vi "nanocal -- nuclear schottky fit V1.vi"() -> ()   [LabVIEW 2020]
uses:
  filename-pattern.ctl
  show-win- control.ctl
  cursor winow.ctl
  cursor window action.ctl
  publisher action.ctl
  3-lorentzian-heat-response action.ctl
  cursor action.ctl
  2Dwindow.ctl
  file -- read-write control.ctl
  array -- freq-voltage transformations action.ctl
  KM_file -- read-write control.ctl
  filename-action.ctl
  9f1323b6-517a-3445-a4b9-7a47222562ae.vi
  3-lorentzian-heat-response.vi/142dd4c5-f9ed-c64b-bc14-a88e3e2c450a.vi
  <vilib>/Analysis/baseanly.llb/A x B.vi
  <vilib>/Analysis/baseanly.llb/Complex A x B.vi
  Q -- check range -- i -- real.vi
  line -- complex.vi
  Q -- check range -- i -- integer.vi
  array -- freq-voltage transformations.vi/05c44075-957c-bc42-b6fa-2799d0bc0485.vi
  Q - not nan -- real.vi
  Q - not nan -- integer.vi
  <vilib>/Array/Sort 2D Array - Pop Stack.vi
  <vilib>/Array/Sort 2D Array - Push Stack.vi
  array -- freq-voltage transformations.vi/05c44075-957c-bc42-b6fa-2799d0bc0485.vi/5dd0d2be-718e-c148-b8fa-e083cdba2843.vi
  array -- freq-voltage transformations.vi/05c44075-957c-bc42-b6fa-2799d0bc0485.vi/095795a0-771d-c341-9fed-d90d2e44c51c.vi
  <vilib>/Analysis/Matrix/Numeric/Conversions/Array To Matrix.vi
  <vilib>/Analysis/Matrix/Numeric/Conversions/Array To Matrix - RA2.vi
  <vilib>/Analysis/baseanly.llb/Inverse Matrix.vi
  <vilib>/Analysis/baseanly.llb/Real Inverse Matrix.vi
  <vilib>/Analysis/polynomials.llb/Multiply Polynomials.vi
  <vilib>/Analysis/polynomials.llb/Multiply Polynomials (DBL).vi
  <vilib>/Analysis/polynomials.llb/Polynomial Roots.vi
  <vilib>/Analysis/polynomials.llb/Polynomial Roots (DBL).vi
  <vilib>/Comparison/Less/Less Functor/Less Functor.lvclass
  server talkto message type.ctl
panel:
  in  "T (K)":dbl=0.001 format="%#_10f"
  out "Plot:  colors":cluster{"Freq out (Hz)":dbl[], dbl[]}[](graph)
  out "String":string
  in  "omega range min (Hz)":dbl=0.001 format="%#_10f"
  in  "omega range max (Hz)":dbl=10000.0 format="%#_10f"
  in  "number of freq points":i32=500
  in  "kappa0":dbl(slide)=5.58e-10 min=0.0 max=0.3 step=1e-12 scale=1e-10..1e-06 scale format="%#_3p"
  in  "tauC":dbl(slide)=0.0059759999999999995 min=0.0 max=0.3 step=1e-06 scale=0.001..10.0 scale format="%#_3p"
  in  "tauN":dbl(slide)=2.349673 min=0.0 max=0.3 step=1e-06 scale=0.001..10.0 scale format="%#_3p"
  in  "tauS":dbl(slide)=0.24445899999999998 min=0.0 max=0.3 step=1e-06 scale=0.001..10.0 scale format="%#_3p"
  in  "T1":dbl(slide)=0.26762 min=0.0 max=0.3 step=1e-06 scale=0.001..10.0 scale format="%#_3p"
  in  "zeta":dbl(slide)=0.23496699999999998 min=0.0 max=0.3 step=1e-06 scale=0.01..10.0 scale format="%#_3p"
  in  "scale gauge: Plot: complex plane":dbl(slide)=625294874.6755459 min=0.0 max=0.3 step=1e-06 scale=1e-05..5000000000.0 scale format="%#_3p"
  in  "Read from file :l":bool
  in  "tr":T1(ring)
  in  "Read from file":path=path "/opt/new/Dropbox/shared_AkashAndreas/paper-CeCoIn5/labviewreadydata/CeCoIn5_2nd_071_12T_0.120K_90deg_fdep_labview_.dat"
  in  "sweeper panel":T2(tab)
  in  ":sweep is ON":bool
  in  "win":T3={"cen (Hz)"=21978.24682616816, "win (Hz)"=4484.832860239923, "left (Hz)"=19735.8303960482, "right (Hz)"=24220.66325628812}
  out "Plot: sweep window":cluster{"Freq out (Hz)":dbl[], dbl[]}[](graph)
  in  "subtract bgnd!":bool
  in  "fit!":bool=TRUE
  in  "cursor window":T4={"left"=19735.8303960482, "right "=24220.66325628812, "center"=21978.24682616816, "window"=4484.832860239923, "cursors"=[0, 1, 2], "relative"=0, "absolute"=0, "fixed vertical offset"=0.0, "vertical offset"=0.0, "skew"=0.0, "default window frac"=0.1, "kind"=enum."symmetric", "skew.left"=0.5, "skew.right"=0.5, "Plot ref"=refnum, "wing order"=enum."forw"}
  in  "save data":enum32{"save/read"}(tab)
  in  "Save to file :s":bool
  in  "Freq sweep name template":T5={"prefix"="RuCl3-rod", "group"="f"}
  in  "Save folder":path=path "/opt/data"
  in  "freq sweep file name":string="f004_RuCl3-rod_060221.dat"
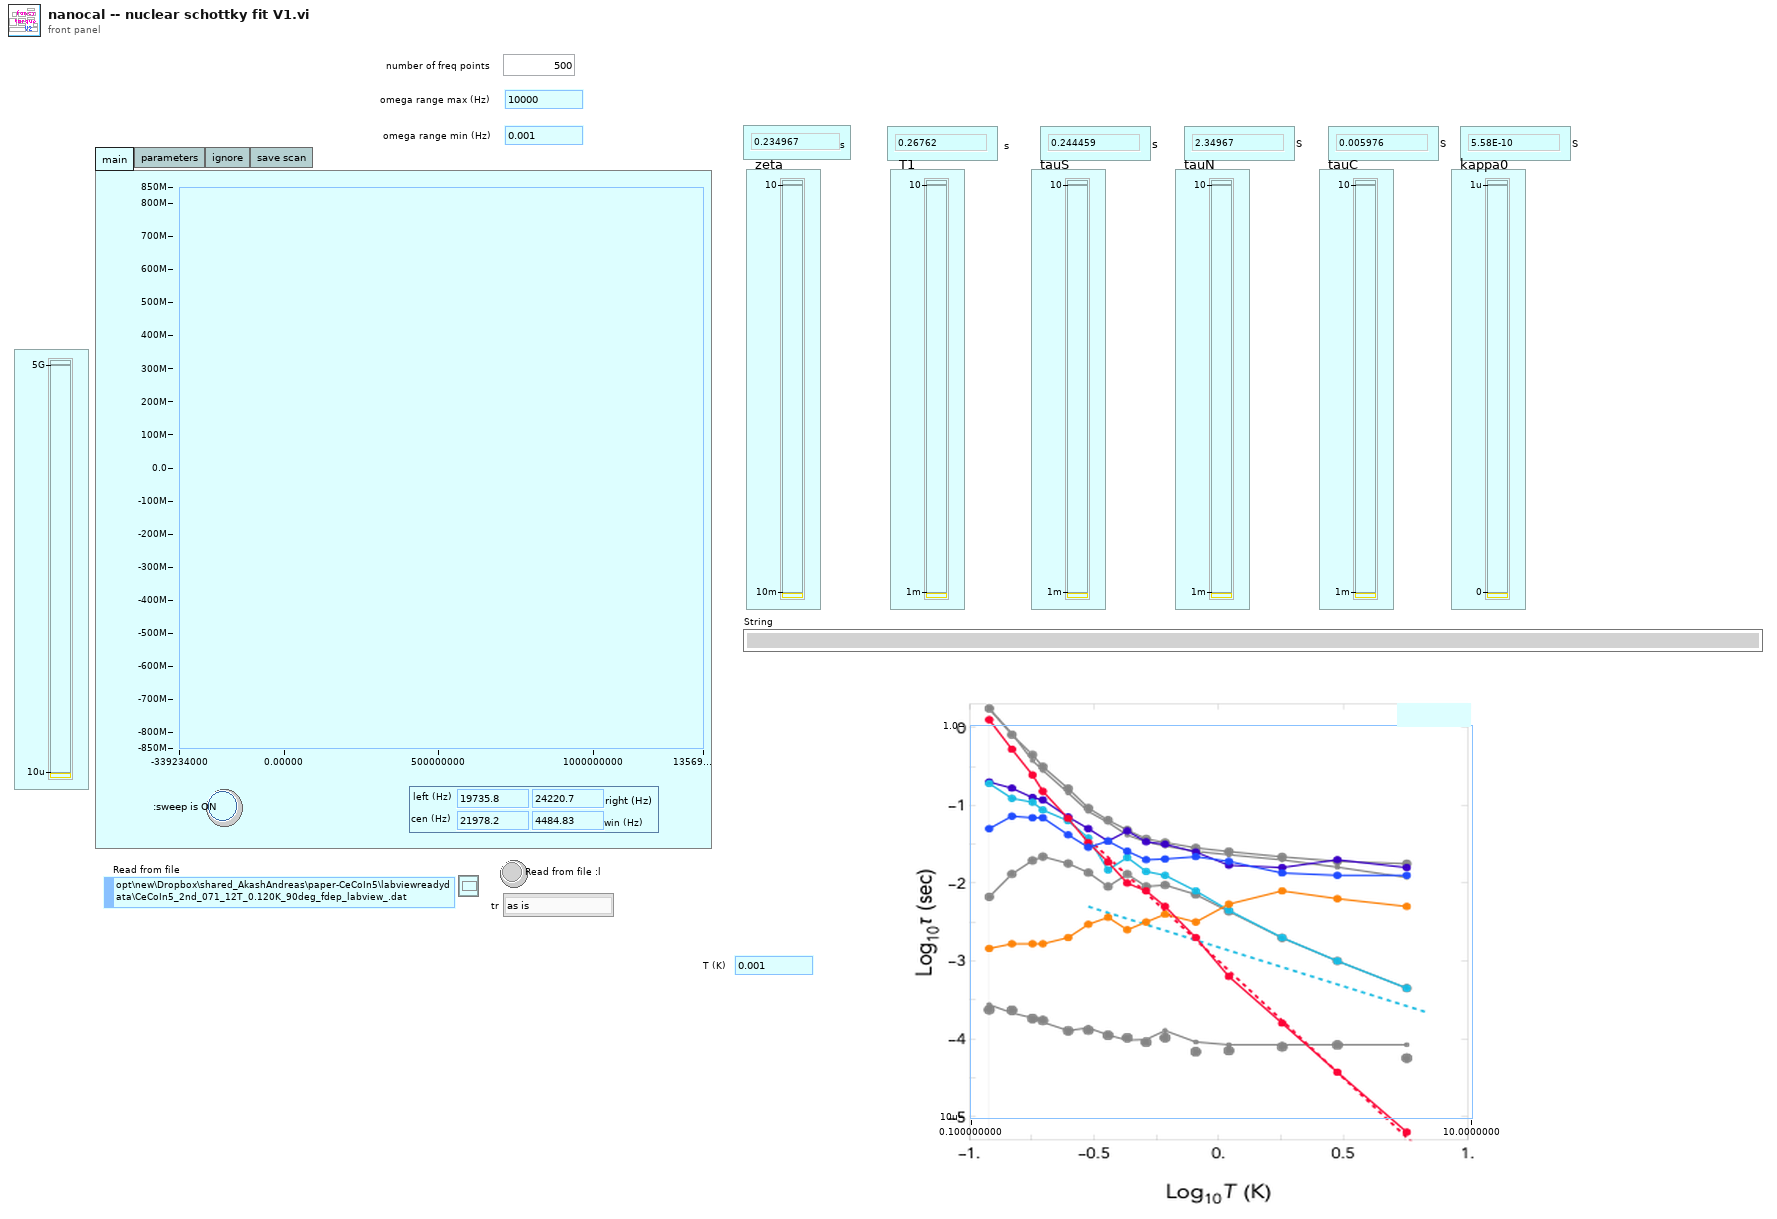
[diagram p1: front panel]
types:
  T1 = enum16{"as is", "add negative freq", "full rydh"}
  T2 = enum32{"main", "parameters", "ignore", "save scan"}
  T3 = typedef "show-win- control.ctl" = cluster{"cen (Hz)":dbl, "win (Hz)":dbl, "left (Hz)":dbl, "right (Hz)":dbl}
  T4 = typedef "cursor winow.ctl" = cluster{"left":dbl, "right ":dbl, "center":dbl, "window":dbl, "cursors":i32[], "relative":i32, "absolute":i32, "fixed vertical offset":dbl, "vertical offset":dbl, "skew":dbl, "default window frac":dbl, "kind":enum16{"symmetric", "skewed", "fancy"}, "skew.left":dbl, "skew.right":dbl, "Plot ref":refnum<vi>, "wing order":enum16{"forw", "back"}}
  T5 = typedef "filename-pattern.ctl" = cluster{"prefix":string, "group":string}
  T6 = typedef "cursor window action.ctl" = enum16{"balance", "h. offset change", "cursor moves", "change center", "change window", "init", "check", "reset", "set y to middle", "idle", "-write all Y", "-write left.X", "-write center.X", "-write right.X", "-write all X", "-change center", "-change window", "-change skew", "-read cursor 2", "-read cursor 1", "-read cursor 0", "-read all cursors", "-reset", "-read plot scale", "-set y to middle", "-Q: center.Y is visible", "-Q: window is visible", "-parse center.Y", "-right left from center", "-left move", "-right move", "-set center.Y", "-empty", "-set cursors to default", "-check", "-write center.Y", "-copy cursor 1", "-copy cursor 0", "-copy cursor 2", "move right", "move left", "shrink", "broaden", "skew up", "skew down", "-write plot scale", "zoom X", "change cen&win", "zoom to all data", "color--red", "color--green", "color--yellow", "read", "zoom out", "zoom in", "slide right", "slide left", "set range aspect ratio to 1"}
  T7 = typedef "3-lorentzian-heat-response action.ctl" = enum16{"calculate response", "create string", "calulate m1m2m3"}
  T8 = typedef "publisher action.ctl" = enum16{"set", "get", "init", "check"}
  T9 = typedef "cursor action.ctl" = enum16{"range", "read", "write", "check", "zoom out", "smart zoom out", "zoom to aspect ratio 1", "zoom to win", "zoom out 20%", "zoom in 20%", "-empty", "smart zoom out&aspect", "move range left 20%", "move range right 20%", "move range up 20%", "move range down 20%", "zoom to X win", "zoom to Y win", "zoom out X", "zoom out Y", "zoom in X", "zoom in Y", "check plot scale"}
  T10 = typedef "2Dwindow.ctl" = cluster{"window y":dbl, "center x":dbl, "center y":dbl, "window x":dbl}
  T11 = typedef "file -- read-write control.ctl" = enum16{"read", "write all", "append one line"}
  T12 = typedef "array -- freq-voltage transformations action.ctl" = enum16{"as is", "add negative freq", "sort freq", "double freq", "R-phase(deg) to Re-Im"}
  T13 = typedef "filename-action.ctl" = enum16{"rewrite", "parse", "force pattern", "uniquenum"}
  T14 = typedef "KM_file -- read-write control.ctl" = enum16{"read", "write all", "append one line"}
  T15 = typedef "server talkto message type.ctl" = cluster{"message":enum16{"stop", "start", "update pars", "update request", "new", "launch", "exit", "get", "reset", "pause", "unpause"}}
  T16 = typedef "eventvkey.ctl" = enum16{"ASCII", "Enter", "Return", "Shift", "Ctrl", "Alt", "Cmd", "Opt", "Caps", "NumLock", "Clear", "Break", "Up", "Down", "Left", "Right", "Insert", "Delete", "Home", "End", "PageUp", "PageDown", "Escape", "Help", "Pause", "ScrollLock", "F1", "F2", "F3", "F4", "F5", "F6", "F7", "F8", "F9", "F10", "F11", "F12", "F13", "F14", "F15", "F16", "F17", "F18", "F19", "F20", "F21", "F22", "F23", "F24", "Play", "VolumeUp", "VolumeDown", "Mute", "Two Byte Char"}
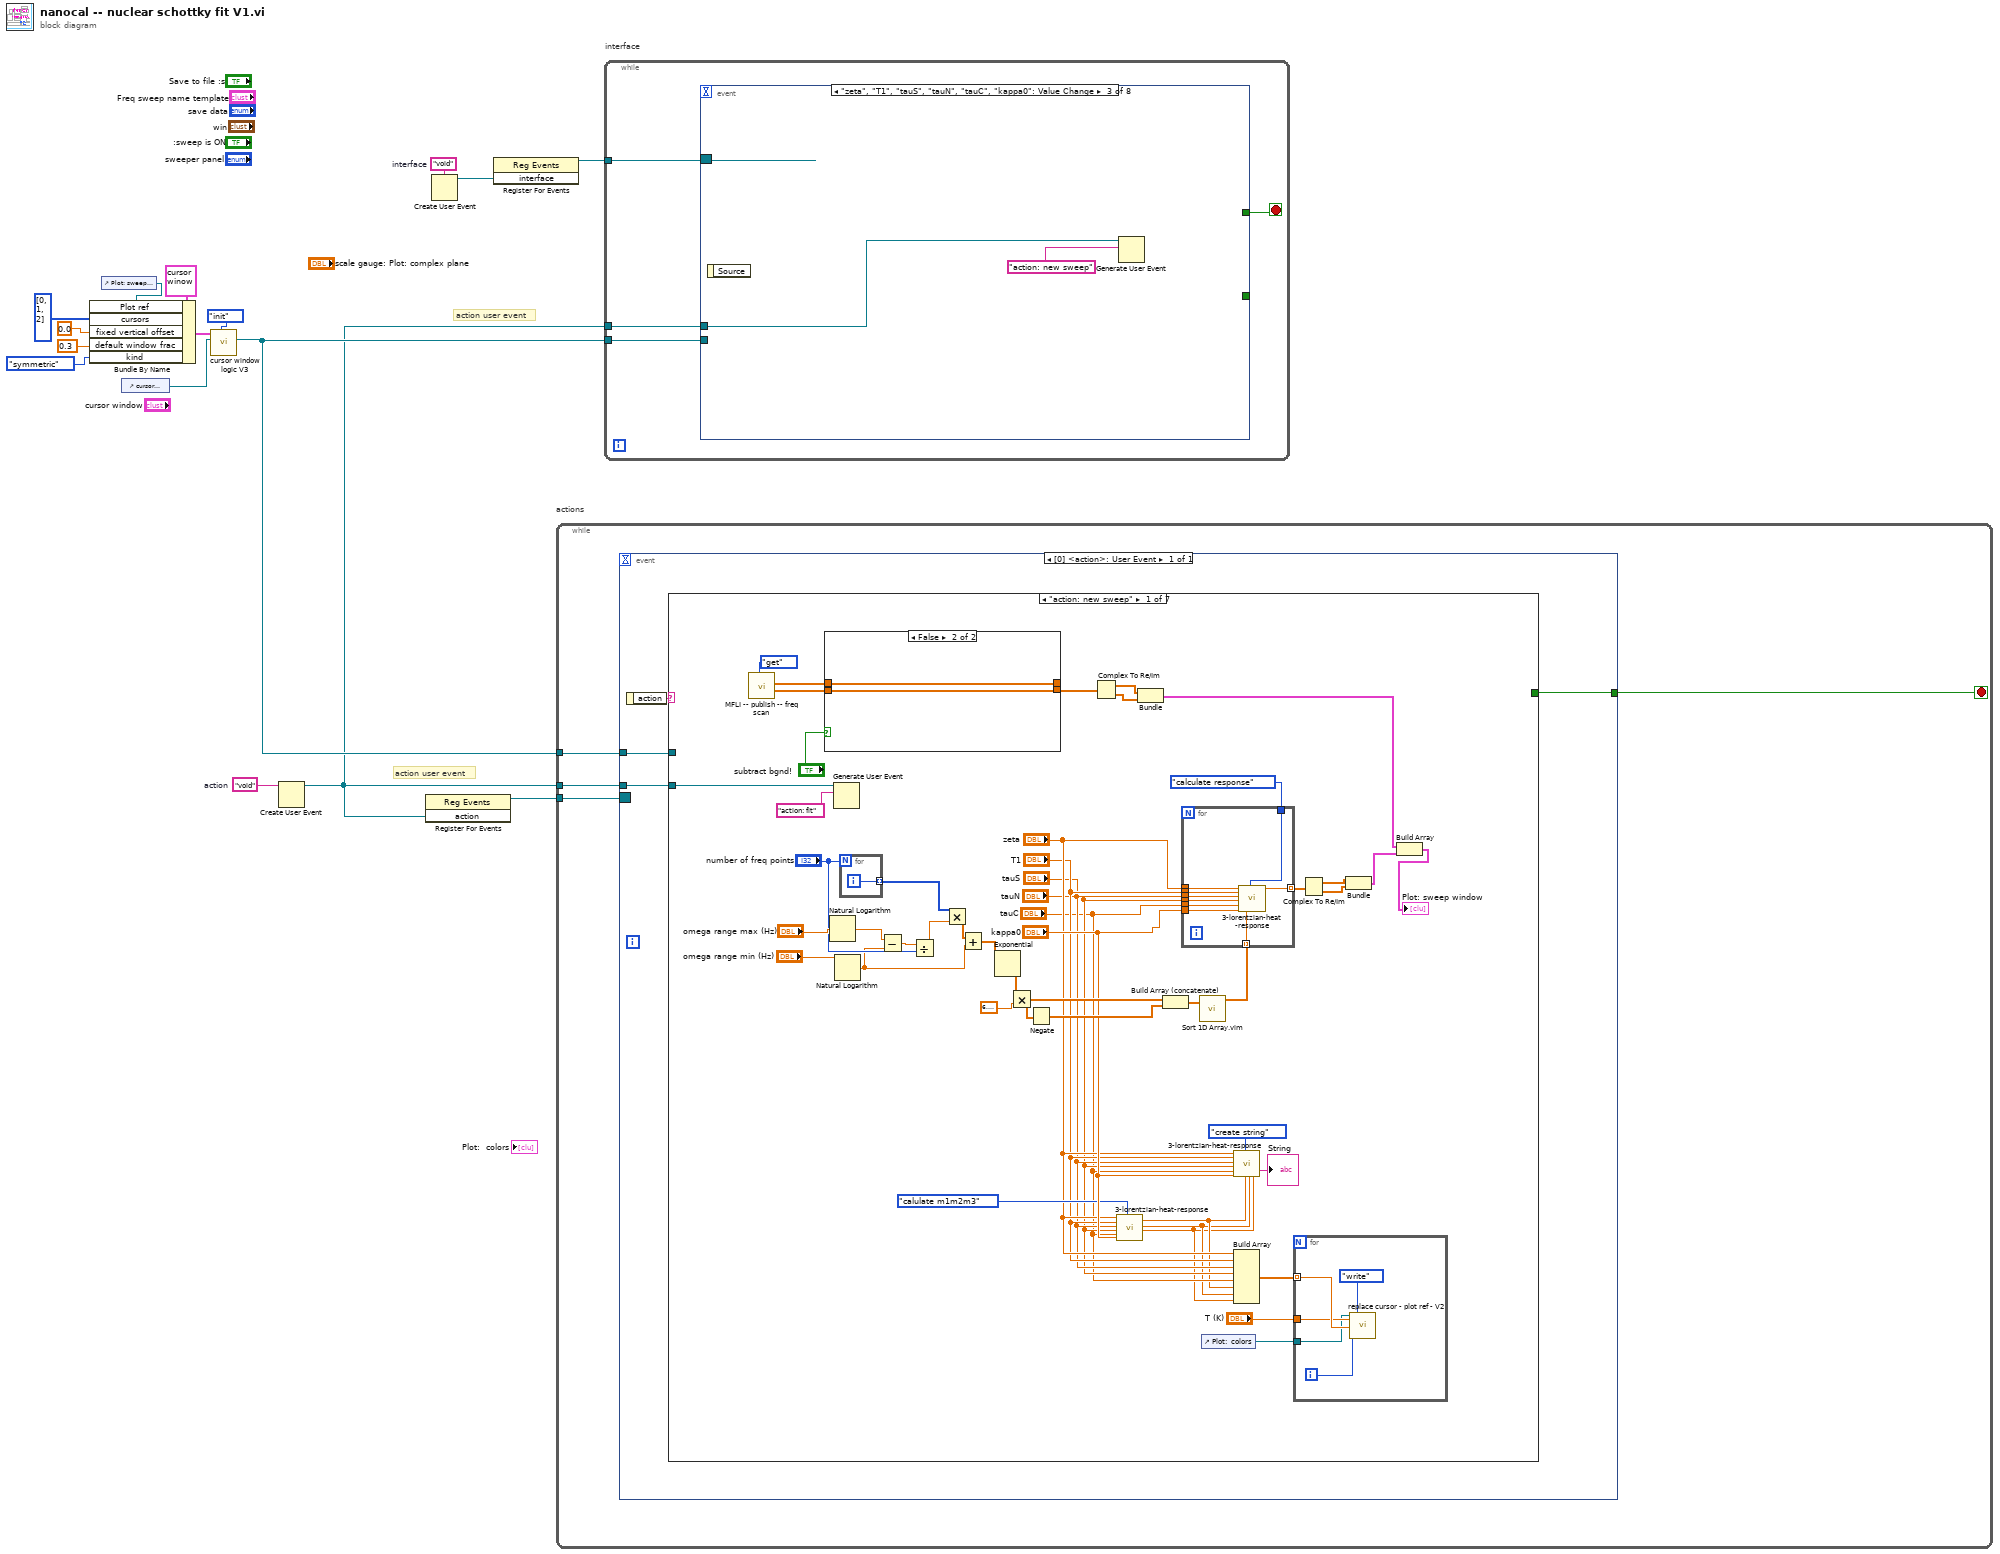
[diagram p0: block diagram]
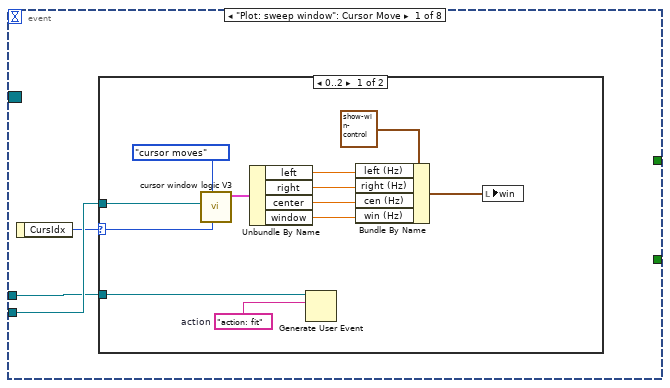
[diagram p2: hidden frame]
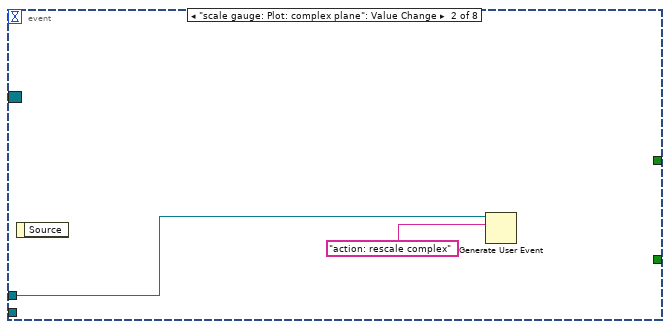
[diagram p4: hidden frame]
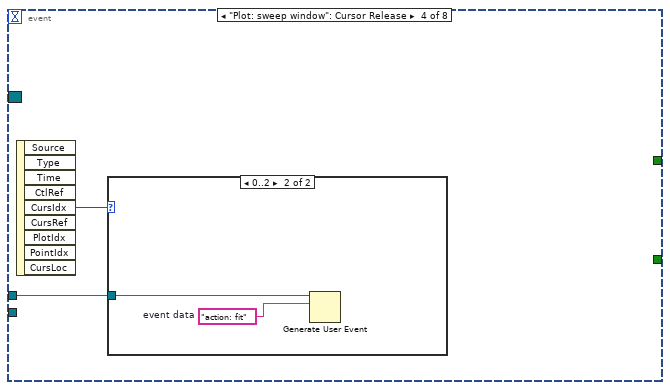
[diagram p5: hidden frame]
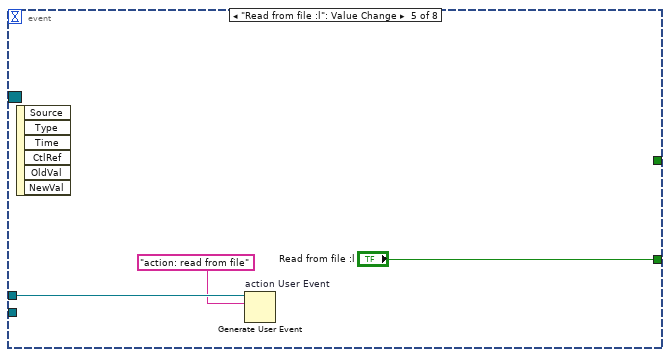
[diagram p7: hidden frame]
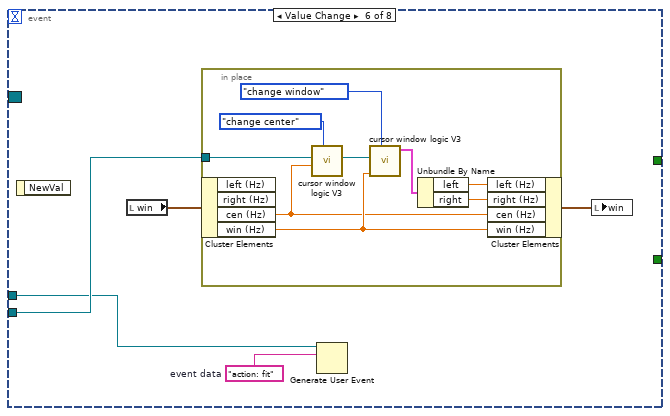
[diagram p8: hidden frame]
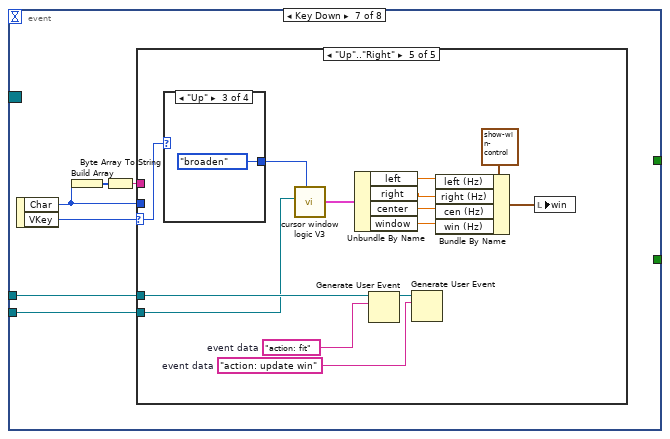
[diagram p9: hidden frame]
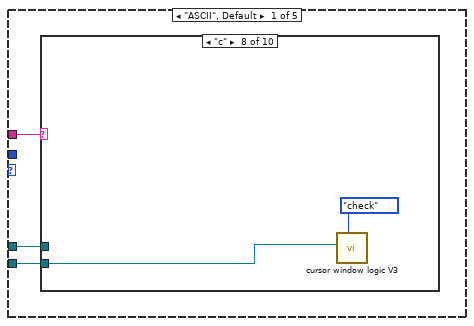
[diagram p10: hidden frame]
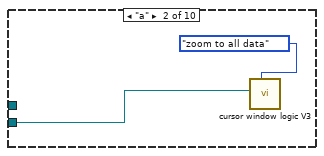
[diagram p12: hidden frame]
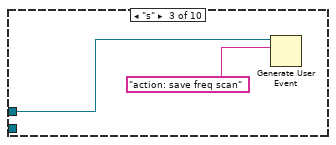
[diagram p13: hidden frame]
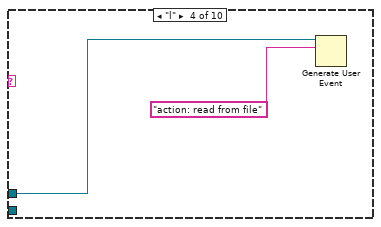
[diagram p14: hidden frame]
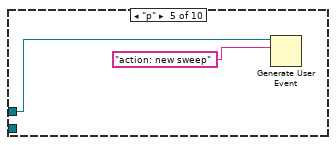
[diagram p15: hidden frame]
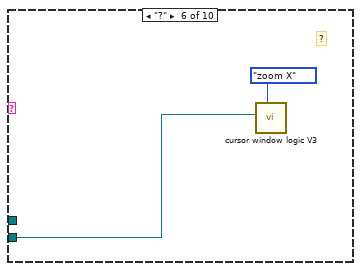
[diagram p16: hidden frame]
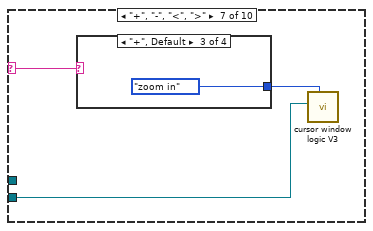
[diagram p17: hidden frame]
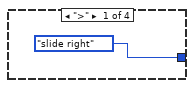
[diagram p18: hidden frame]
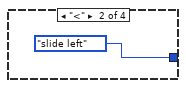
[diagram p19: hidden frame]
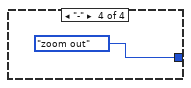
[diagram p20: hidden frame]
diagram:
  w13 = "void"  # interface
  w15 = "void"  # action
  # "action user event"
  # "action user event"
  n1 = control-ref of="Plot: sweep window"() -> (w4:refnum<vi>)
  n2 = Bundle By Name(cluster=T4 {"left"=0.0, "right "=0.0, "center"=0.0, "window"=0.0, "cursors"=[], "relative"=0, "absolute"=0, "fixed vertical offset"=0.0, "vertical offset"=0.0, "skew"=0.0, "default window frac"=0.0, "kind"=enum."symmetric", "skew.left"=0.0, "skew.right"=0.0, "Plot ref"=refnum, "wing order"=enum."forw"} ("cursor bracket: All, data window"), "Plot ref"=w4, "cursors"=i32[] [0, 1, 2], "fixed vertical offset"=0.0, "default window frac"=0.3 ("fixed vertical offset"), "kind"=enum16{"symmetric", "skewed", "fancy"}."symmetric") -> (w8:T4)
  n3 = control-ref of="cursor window"() -> (w3:refnum<vi>)
  n4 = call "cursor window logic V3.vi"("cursor window action"=cursor_window_action."init", "cursor window in"=w3, "cursor window init"=w8) -> ("cursor window out"=w6:refnum<vi>)  [unwired: 7 in, 1 out]
  n5 = Create User Event(user event datatype=w15) -> (user event=w1:refnum<user-event>)  [unwired: 1 in, 1 out]
  n6 = register-events(w1) -> (reference out=w16:refnum<event-registration>)  [unwired: 2 in, 1 out]
  n7 = Create User Event(user event datatype=w13) -> (user event=w2:refnum<user-event>)  [unwired: 1 in, 1 out]
  n8 = register-events(w2) -> (reference out=w14:refnum<event-registration>)  [unwired: 2 in, 1 out]
  n9 = while "actions" {
    tunnel: w16 -> [w20]
    tunnel: w1 -> [w19]
    tunnel: w6 -> [w18]
    stop <- w17 stop-if-true
    n10 = event shown="[0] <action>: User Event" {
      selector: w20 -> [_]
      dyn-events: _ -> [_]
      timeout: _ -> [_]
      tunnel: w19 -> [w23]
      tunnel: w18 -> [w22]
      tunnel: [w21] -> w17
      event User Event {
        n11 = event-data() -> ("action"=w24:string)  [unwired: 1 in]
        n12 = case shown="\"action: new sweep\"" w24 {
          tunnel: w23 -> [w69 _ _ w118 _ _ _]
          tunnel: w22 -> [_ _ _ _ _ w174 _]
          tunnel: [_ _ TRUE _ _ _ _] -> w21
          frame "action: new sweep" {
            n13 = call "MFLI -- publish -- freq scan.vi"("publisher action"=publisher_action."get") -> ("Voltage out (V)"=w67:cdb[], "Freq out (Hz)"=w68:dbl[])  [unwired: 9 in]
            n14 = case shown="False" "subtract bgnd!" {
              tunnel: w68 -> [w94 w102]
              tunnel: [w88 w102] -> _
              tunnel: w67 -> [w90 w101]
              tunnel: [w95 w101] -> w66
              frame True {
                w87 = 10 ("length")
                n15 = Delete From Array(array=w94, length=w87, index=0) -> (array with subset deleted=w93:dbl[])  [unwired: 1 out]
                n16 = Delete From Array(array=w90, length=w87, index=0) -> (array with subset deleted=w89:cdb[])  [unwired: 1 out]
                n17 = call "linear interp iiii- complex - z-omega.vi"("z"=w89, "omega"=w93) -> ("z out"=w96:cdb[], "omega out"=w88:dbl[], "intercept"=w98:cdb, "slope"=w99:cdb)  [unwired: 5 in, 5 out]
                n18 = Multiply(x=w88, y=w99) -> (x*y=w100:cdb[])
                n19 = Add(x=w100, y=w98) -> (x+y=w97:cdb[])
                n20 = Subtract(x=w96, y=w97) -> (x-y=w95:cdb[])
              }
              frame False {
              }
            }
            n21 = Natural Logarithm(1:"omega range max (Hz)") -> (0:w58:dbl)
            n22 = Generate User Event(user event=w69, event data cluster="action: fit" ("event data")) -> ()  [unwired: 2 in, 2 out]
            n23 = Natural Logarithm(1:"omega range min (Hz)") -> (0:w53:dbl)
            n24 = for {
              N: "number of freq points" -> [_]
              tunnel: [w77] -> w55 mode=indexing
              i -> [w77]
            }
            n25 = Subtract(x=w58, y=w53) -> (x-y=w57:dbl)
            n26 = Divide(x=w57, y="number of freq points") -> (x/y=w54:dbl)
            n27 = Multiply(x=w55, y=w54) -> (x*y=w52:dbl[])
            n28 = Add(x=w52, y=w53) -> (x+y=w51:dbl[])
            n29 = Exponential(1:w51) -> (0:w50:dbl[])
            n30 = Multiply(x=w50, y=6.283185307179586) -> (x*y=w44:dbl[])
            n31 = Negate(x=w44) -> (-x=w43:dbl[])
            n32 = Complex To Re/Im(x + iy=w66) -> (x=w61:dbl[], y=w71:dbl[])
            n33 = call "3-lorentzian-heat-response.vi"("zeta"="zeta", "T1"="T1", "tauS"="tauS", "tauN"="tauN", "tauC"="tauC", "kappa0"="kappa0", "action"=3-lorentzian-heat-response_action."calulate m1m2m3") -> ("m1"=w30:dbl, "m2"=w29:dbl, "m3"=w28:dbl)  [unwired: 8 in, 2 out]
            n34 = Bundle(w61, w71) -> (w70:cluster{dbl[], dbl[]})  [unwired: 1 in]
            n35 = Build Array (concatenate)(w44, w43) -> (w42:dbl[])
            n36 = call "Sort 1D Array.vim"("unsorted array"=w42) -> ("sorted array"=w41:dbl[])  [unwired: 10 in]
            n37 = for {
              tunnel: "zeta" -> [w86]
              tunnel: "T1" -> [w85]
              tunnel: "tauS" -> [w84]
              tunnel: "tauN" -> [w83]
              tunnel: "tauC" -> [w82]
              tunnel: "kappa0" -> [w81]
              tunnel: w41 -> [w80] mode=indexing
              tunnel: [w79] -> w48 mode=indexing
              tunnel: 3-lorentzian-heat-response_action."calculate response" ("action") -> [w78]
              n38 = call "3-lorentzian-heat-response.vi"("zeta"=w86, "T1"=w85, "tauS"=w84, "tauN"=w83, "tauC"=w82, "kappa0"=w81, "omega (rad)"=w80, "action"=w78) -> ("Romega"=w79:cdb)  [unwired: 7 in, 4 out]
            }
            n39 = control-ref of="Plot:  colors"() -> (w25:refnum<vi>)
            n40 = call "3-lorentzian-heat-response.vi"("zeta"="zeta", "T1"="T1", "tauS"="tauS", "tauN"="tauN", "tauC"="tauC", "kappa0"="kappa0", "action"=3-lorentzian-heat-response_action."create string", "m1 IN"=w30, "m2 IN"=w29, "m3 IN"=w28) -> ("String"=→"String":string)  [unwired: 5 in, 4 out]
            n41 = Build Array("zeta", "T1", "tauS", "tauN", "tauC", w30, w29, w28) -> (w27:dbl[])
            n42 = for {
              tunnel: w27 -> [w76] mode=indexing
              tunnel: "T (K)" -> [w75]
              tunnel: w25 -> [w73]
              i -> [w72]
              n43 = call "replace cursor - plot ref - V2.vi"("Plot ref in"=w73, "new X"=w75, "new  Y"=w76, "cursor index"=w72, "cursor action"=cursor_action."write") -> ()  [unwired: 11 in, 4 out]
            }
            n44 = Complex To Re/Im(x + iy=w48) -> (x=w47:dbl[], y=w46:dbl[])
            n45 = Bundle(w47, w46) -> (w45:cluster{dbl[], dbl[]})  [unwired: 1 in]
            n46 = Build Array(w70, w45) -> (→"Plot: sweep window":cluster{dbl[], dbl[]}[])
          }
          frame "action: rescale complex" {
            n47 = local read "scale gauge: Plot: complex plane"() -> (w105:dbl)
            n48 = control-ref of="Plot: sweep window"() -> (w107:refnum<vi>)
            n49 = Multiply(x=w105, y=0.3) -> (x*y=w103:dbl)
            n50 = Bundle By Name(cluster=T10 {"window y"=0.0021014740628288917, "center x"=44850.89441339177, "center y"=2.5658109925320947, "window x"=17480.201988350764} ("window IN"), "window x"=w105, "window y"=w105, "center x"=w103, "center y"=0.0) -> (w110:T10)
            n51 = call "replace cursor - plot ref - V2.vi"("Plot ref in"=w107, "window IN"=w110, "cursor action"=cursor_action."zoom to win") -> ()  [unwired: 13 in, 4 out]
          }
          frame "action: exit" {
            n52 = local write ":sweep is ON"(FALSE ("sweep ON")) -> ()
          }
          frame "action: read from file" {
            n53 = call "file - read-write - list of lines.vi"("read/write control"=file_--_read-write_control."read", "file path"="Read from file") -> ("list of lines OUT"=w122:string[])  [unwired: 8 in, 1 out]
            n54 = for {
              tunnel: w122 -> [w157] mode=indexing
              tunnel: [w152] -> w117 mode=indexing if=w148
              tunnel: [w151] -> w116 mode=indexing if=w148
              w153 = 0.0
              n55 = Scan From String(format string="%f%f%f", input string=w157, initial scan location=u32 0, default 1=w153, default 2=w153, default 3=w153) -> (offset past scan=w149:u32, output 1=w151:dbl, output 2=w155:dbl, output 3=w154:dbl)  [unwired: 1 in, 2 out]
              n56 = Greater Than 0?(x=w149) -> (x > 0?=w148:bool)
              n57 = Re/Im To Complex(1:w154, 2:w155) -> (0:w152:cdb)
            }
            n58 = case shown="\"add negative freq\"" "tr" {
              tunnel: w117 -> [w124 w126 w138]
              tunnel: w116 -> [w125 w133 w147]
              tunnel: [w125 w130 w144] -> w114
              tunnel: [w124 w129 w143] -> w113
              frame "as is", Default {
              }
              frame "add negative freq" {
                n59 = call "array -- freq-voltage transformations.vi"("freq voltage action"=array_--_freq-voltage_transformations_action."add negative freq", "z In"=w126, "freq IN"=w133) -> ("z out"=w131:cdb[], "freq out"=w132:dbl[])  [unwired: 7 in]
                n60 = call "array -- freq-voltage transformations.vi"("freq voltage action"=array_--_freq-voltage_transformations_action."sort freq", "z In"=w131, "freq IN"=w132) -> ("z out"=w129:cdb[], "freq out"=w130:dbl[])  [unwired: 7 in]
              }
              frame "full rydh" {
                n61 = call "array -- freq-voltage transformations.vi"("freq voltage action"=array_--_freq-voltage_transformations_action."double freq", "z In"=w138, "freq IN"=w147) -> ("z out"=w137:cdb[], "freq out"=w140:dbl[])  [unwired: 7 in]
                n62 = call "array -- freq-voltage transformations.vi"("freq voltage action"=array_--_freq-voltage_transformations_action."R-phase(deg) to Re-Im", "z In"=w137, "freq IN"=w140) -> ("z out"=w136:cdb[], "freq out"=w139:dbl[])  [unwired: 7 in]
                n63 = call "array -- freq-voltage transformations.vi"("freq voltage action"=array_--_freq-voltage_transformations_action."add negative freq", "z In"=w136, "freq IN"=w139) -> ("z out"=w145:cdb[], "freq out"=w146:dbl[])  [unwired: 7 in]
                n64 = call "array -- freq-voltage transformations.vi"("freq voltage action"=array_--_freq-voltage_transformations_action."sort freq", "z In"=w145, "freq IN"=w146) -> ("z out"=w143:cdb[], "freq out"=w144:dbl[])  [unwired: 7 in]
              }
            }
            n65 = flat-sequence {
              tunnel: w118 -> [w161]
              tunnel: [w161] -> w123
              tunnel: w113 -> [w159]
              tunnel: w114 -> [w158]
              tunnel: w123 -> [w163]
              tunnel: "action: new sweep" ("event data") -> [w162]
              frame #0 {
                n66 = call "MFLI -- publish -- freq scan.vi"("publisher action"=publisher_action."set", "Voltage IN (V)"=w159, "Freq IN (Hz)"=w158) -> ()  [unwired: 7 in, 2 out]
              }
              frame #1 {
                n67 = Generate User Event(user event=w163, event data cluster=w162) -> ()  [unwired: 2 in, 2 out]
              }
            }
          }
          frame "action: save freq scan" {
            n68 = local read "Freq sweep name template"() -> (w169:T5)
            n69 = call "MFLI -- publish -- freq scan.vi"("publisher action"=publisher_action."get") -> ("Voltage out (V)"=w165:cdb[], "Freq out (Hz)"=w166:dbl[])  [unwired: 9 in]
            n70 = call "filename-manage.vi"("filename pattern"=w169, "filename-action"=filename-action."uniquenum", "folder"="Save folder", "file name"="freq sweep file name") -> ("filename OUT"=w168:string)  [unwired: 7 in]
            n71 = call "KM_appendline -- freq sweep.vi"("freq"=w166, "Vout(V)"=w165, "Save frequency scan"="Save folder", "read/write control"=KM_file_--_read-write_control."append one line", "name or relative path"=w168) -> ()  [unwired: 15 in]
            n72 = local write "freq sweep file name"(w168) -> ()
          }
          frame "action: fit" {
            n73 = case shown="True" "fit!" {
              tunnel: w174 -> [_ w175]
              frame False {
              }
              frame True {
                n74 = flat-sequence {
                  tunnel: w175 -> [w178]
                  frame #0 {
                    n75 = call "cursor window logic V3.vi"("cursor window action"=cursor_window_action."read", "cursor window in"=w178) -> ("cursor window out"=w177:T4)  [unwired: 8 in, 1 out]
                    n76 = call "publish -- fitter window.vi"("publisher action"=publisher_action."set", "win IN"=w177) -> ()  [unwired: 9 in, 1 out]
                  }
                  frame #1 {
                    n77 = disable-structure shown="Disabled" {
                      frame Disabled {
                        n78 = Generate User Event(event data cluster=T15 {"message"=enum."new"} ("event data")) -> ()  [unwired: 3 in, 2 out]
                      }
                      frame Enabled {
                      }
                    }
                  }
                }
              }
            }
          }
          frame "void", Default {
          }
        }
      }
    }
  }
  n79 = while "interface" {
    tunnel: w14 -> [w184]
    tunnel: w1 -> [w183]
    tunnel: w6 -> [w182]
    stop <- w181 stop-if-true
    n80 = event shown="[2] \"zeta\", \"T1\", \"tauS\", \"tauN\", \"tauC\", \"kappa0\": Value Change" {
      selector: w184 -> [_ _ _ _ _ _ _ _]
      dyn-events: _ -> [_ _ _ _ _ _ _ _]
      timeout: _ -> [_ _ _ _ _ _ _ _]
      tunnel: w183 -> [w185 w200 w202 w205 w210 w211 w229 _]
      tunnel: w182 -> [w187 _ _ _ _ w215 w225 _]
      tunnel: [_ _ _ _ "Read from file :l" _ _ _] -> _
      tunnel: [_ _ _ _ _ _ _ w273] -> w181
      event "Plot: sweep window": Cursor Move {
        n81 = event-data() -> ("CursIdx"=w186:i32)  [unwired: 1 in]
        n82 = case shown="0..2" w186 {
          selector: w186 -> [w197 _]
          tunnel: w187 -> [w199 _]
          tunnel: w185 -> [w195 _]
          frame 0..2 {
            w194 = "action: fit"  # action
            n83 = call "cursor window logic V3.vi"("CursIdx"=w197, "cursor window action"=cursor_window_action."cursor moves", "cursor window in"=w199) -> ("cursor window out"=w196:T4)  [unwired: 7 in, 1 out]
            n84 = Unbundle By Name(w196) -> ("left"=w191:dbl, "right"=w190:dbl, "center"=w189:dbl, "window"=w188:dbl)
            n85 = Generate User Event(user event=w195, event data cluster=w194) -> ()  [unwired: 2 in, 2 out]
            n86 = Bundle By Name(cluster=T3 {"cen (Hz)"=-0.35260838541595674, "win (Hz)"=17.234446484426172, "left (Hz)"=-8.969831627629043, "right (Hz)"=8.26461485679713} ("win"), "left (Hz)"=w191, "right (Hz)"=w190, "cen (Hz)"=w189, "win (Hz)"=w188) -> (w192:T3)
            n87 = local write "win"(w192) -> ()
          }
          frame 3..5, Default {
          }
        }
      }
      event "scale gauge: Plot: complex plane": Value Change {
        n88 = event-data() -> ()  [unwired: 1 in, 1 out]
        n89 = Generate User Event(user event=w200, event data cluster="action: rescale complex" ("event data")) -> ()  [unwired: 2 in, 2 out]
      }
      event "zeta", "T1", "tauS", "tauN", "tauC", "kappa0": Value Change {
        n90 = event-data() -> ()  [unwired: 1 in, 1 out]
        n91 = Generate User Event(user event=w202, event data cluster="action: new sweep" ("event data")) -> ()  [unwired: 2 in, 2 out]
      }
      event "Plot: sweep window": Cursor Release {
        n92 = event-data() -> ("CursIdx"=w204:i32)  [unwired: 1 in, 8 out]
        n93 = case shown="0..2" w204 {
          tunnel: w205 -> [_ w206]
          frame 3, Default {
          }
          frame 0..2 {
            w207 = "action: fit"  # event data
            n94 = Generate User Event(user event=w206, event data cluster=w207) -> ()  [unwired: 2 in, 2 out]
          }
        }
      }
      event "Read from file :l": Value Change {
        n95 = event-data() -> ()  [unwired: 1 in, 6 out]
        n96 = Generate User Event "action User Event"(user event=w210, event data cluster="action: read from file" ("event data")) -> ()  [unwired: 2 in, 2 out]
      }
      event Value Change {
        w212 = "action: fit"  # event data
        n97 = event-data() -> ()  [unwired: 1 in, 1 out]
        n98 = local read "win"() -> (w214:T3)
        n99 = in-place {
          in-place-border: w215 -> [w221]
          n100 = in-place-cluster #1(w214) -> ("cen (Hz)"=w216:dbl, "win (Hz)"=w217:dbl)  [unwired: 2 out]
          n101 = call "cursor window logic V3.vi"("cursor window action"=cursor_window_action."change center", "center"=w216, "cursor window in"=w221) -> ("cursor window out"=w222:refnum<vi>)  [unwired: 7 in, 1 out]
          n102 = call "cursor window logic V3.vi"("cursor window action"=cursor_window_action."change window", "window"=w217, "cursor window in"=w222) -> ("cursor window out"=w220:T4)  [unwired: 7 in, 1 out]
          n103 = Unbundle By Name(w220) -> ("left"=w219:dbl, "right"=w218:dbl)
          n104 = in-place-cluster #1("left (Hz)"=w219, "right (Hz)"=w218, "cen (Hz)"=w216, "win (Hz)"=w217) -> (w213:T3)
        }
        n105 = Generate User Event(user event=w211, event data cluster=w212) -> ()  [unwired: 2 in, 2 out]
        n106 = local write "win"(w213) -> ()
      }
      event Key Down {
        n107 = event-data() -> ("Char"=w227:i16, "VKey"=w230:T16)  [unwired: 1 in]
        n108 = Build Array(w227) -> (w228:i16[])
        n109 = Byte Array To String(unsigned byte array=w228) -> (string=w226:string)
        n110 = case shown="\"Up\"..\"Right\"" w230 {
          selector: w230 -> [_ _ _ _ w268]
          tunnel: w227 -> [_ _ _ _ _]
          tunnel: w229 -> [w233 _ _ _ w267]
          tunnel: w226 -> [w232 _ _ _ _]
          tunnel: w225 -> [w231 _ _ _ w264]
          frame "ASCII", Default {
            n111 = case shown="\"c\"" w232 {
              selector: w232 -> [_ _ _ _ _ _ w245 _ _ _]
              tunnel: w233 -> [_ _ w236 w238 w240 _ _ _ _ w254]
              tunnel: w231 -> [_ w234 _ _ _ w242 w246 w251 _ _]
              frame "0", Default {
              }
              frame "a" {
                n112 = call "cursor window logic V3.vi"("cursor window action"=cursor_window_action."zoom to all data", "cursor window in"=w234) -> ()  [unwired: 8 in, 2 out]
              }
              frame "s" {
                n113 = Generate User Event(user event=w236, event data cluster="action: save freq scan" ("event data")) -> ()  [unwired: 2 in, 2 out]
              }
              frame "l" {
                n114 = Generate User Event(user event=w238, event data cluster="action: read from file" ("event data")) -> ()  [unwired: 2 in, 2 out]
              }
              frame "p" {
                n115 = Generate User Event(user event=w240, event data cluster="action: new sweep" ("event data")) -> ()  [unwired: 2 in, 2 out]
              }
              frame "?" {
                # "?"
                n116 = call "cursor window logic V3.vi"("cursor window action"=cursor_window_action."zoom X", "cursor window in"=w242) -> ()  [unwired: 8 in, 2 out]
              }
              frame "+", "-", "<", ">" {
                n117 = case shown="\"+\", Default" w245 {
                  tunnel: [cursor_window_action."slide right" ("cursor window action") cursor_window_action."slide left" ("cursor window action") cursor_window_action."zoom in" ("cursor window action") cursor_window_action."zoom out" ("cursor window action")] -> w244
                  frame ">" {
                  }
                  frame "<" {
                  }
                  frame "+", Default {
                  }
                  frame "-" {
                  }
                }
                n118 = call "cursor window logic V3.vi"("cursor window action"=w244, "cursor window in"=w246) -> ()  [unwired: 8 in, 2 out]
              }
              frame "c" {
                n119 = call "cursor window logic V3.vi"("cursor window action"=cursor_window_action."check", "cursor window in"=w251) -> ()  [unwired: 8 in, 2 out]
              }
              frame "t" {
              }
              frame "r" {
                n120 = Generate User Event(user event=w254, event data cluster="action: toggle sweep!" ("event data")) -> ()  [unwired: 2 in, 2 out]
              }
            }
          }
          frame "Escape" {
          }
          frame "PageUp" {
          }
          frame "PageDown" {
          }
          frame "Up".."Right" {
            w255 = "action: update win"  # event data
            w257 = "action: fit"  # event data
            n121 = case shown="\"Up\"" w268 {
              tunnel: [cursor_window_action."move right" ("cursor window action") cursor_window_action."move left" ("cursor window action") cursor_window_action."broaden" ("cursor window action") cursor_window_action."shrink" ("cursor window action")] -> w266
              frame "Right", Default {
              }
              frame "Left" {
              }
              frame "Up" {
              }
              frame "Down" {
              }
            }
            n122 = call "cursor window logic V3.vi"("cursor window action"=w266, "cursor window in"=w264) -> ("cursor window out"=w265:T4)  [unwired: 8 in, 1 out]
            n123 = Unbundle By Name(w265) -> ("left"=w261:dbl, "right"=w260:dbl, "center"=w259:dbl, "window"=w258:dbl)
            n124 = Generate User Event(user event=w267, event data cluster=w257) -> (user event out=w256:refnum<user-event>)  [unwired: 2 in, 1 out]
            n125 = Generate User Event(user event=w256, event data cluster=w255) -> ()  [unwired: 2 in, 2 out]
            n126 = Bundle By Name(cluster=T3 {"cen (Hz)"=-0.35260838541595674, "win (Hz)"=17.234446484426172, "left (Hz)"=-8.969831627629043, "right (Hz)"=8.26461485679713} ("win"), "left (Hz)"=w261, "right (Hz)"=w260, "cen (Hz)"=w259, "win (Hz)"=w258) -> (w263:T3)
            n127 = local write "win"(w263) -> ()
          }
        }
      }
      event User Event {
        n128 = event-data() -> ("interface"=w274:string)  [unwired: 1 in, 4 out]
        n129 = case shown="\"False\", Default" w274 {
          tunnel: [_ TRUE] -> w273
          frame "False", Default {
          }
          frame "interface: exit" {
          }
        }
      }
    }
  }
